vi "Store UI Ref.vi"(8 "error in (no error)":errorcluster, 11 "Mag Lab Measure Interface in":refnum<class "Mag Lab Measure UI.lvclass">) -> (0 "error out":errorcluster, 3 "Mag Lab Measure Interface out":refnum<class "Mag Lab Measure UI.lvclass">)   [LabVIEW 2015, in "Mag Lab Measure UI.lvclass"]
uses:
  Mag Lab Measure UI.lvclass
  Mag Lab Root/Mag Lab Root.lvclass/Mag Lab Root.ctl
  Mag Lab Measure UI.lvclass/Mag Lab Measure UI.ctl
  Mag Lab Root/Read Front Panel ref.vi
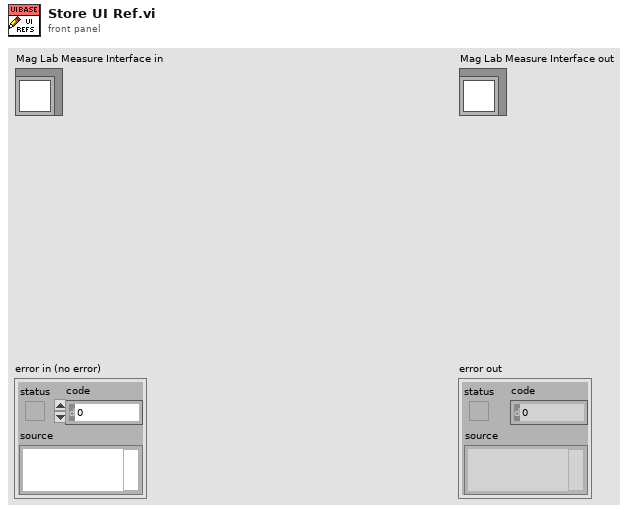
[diagram p1: front panel]
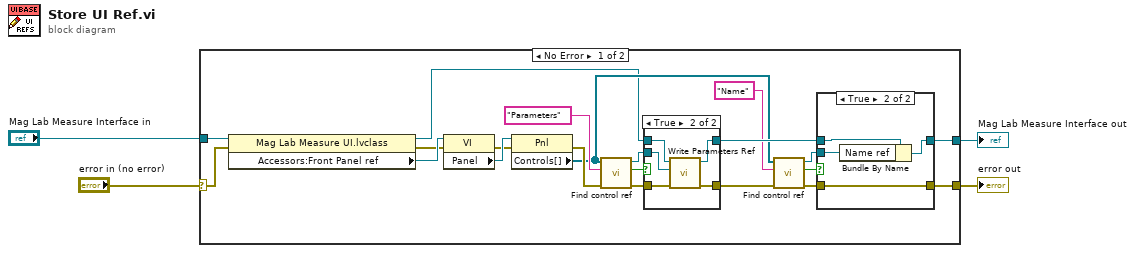
[diagram p0: block diagram]
diagram:
  n1 = case shown="No Error" "error in (no error)" {
    selector: "error in (no error)" -> [w5 w40]
    tunnel: [w16 w40] -> w3
    tunnel: [w17 w39] -> w1
    tunnel: "Mag Lab Measure Interface in" -> [w9 w39]
    frame No Error {
      n2 = property class="Mag Lab Measure UI.lvclass"(reference=w9, error in=w5) -> (reference out=w7:refnum<class "Mag Lab Measure UI.lvclass">, error out=w6:errorcluster, "Accessors:Front Panel ref"=w8:refnum<vi>)
      n3 = property class="VI"(reference=w8, error in=w6) -> (error out=w23:errorcluster, "Panel"=w24:refnum<vi>)  [unwired: 1 out]
      n4 = property class="Pnl"(reference=w24, error in=w23) -> (error out=w25:errorcluster, "Controls[]"=w11:refnum<vi>[])  [unwired: 1 out]
      n5 = call "Find control ref.vi"("error in (no error)"=w25, "Label"="Parameters", "Controls[]"=w11) -> ("error out"=w22:errorcluster, "Found"=w21:bool, "Control out"=w20:refnum<vi>)  [unwired: 6 in]
      n6 = case shown="True" w21 {
        tunnel: w7 -> [w33 w38]
        tunnel: [w33 w37] -> w18
        tunnel: w22 -> [w32 w36]
        tunnel: [w32 w35] -> w14
        tunnel: w20 -> [_ w34]
        frame False {
        }
        frame True {
          n7 = call "Write Parameters Ref.vi"("error in (no error)"=w36, "Parameters"=w34, "Mag Lab Measure Interface in"=w38) -> ("error out"=w35:errorcluster, "Mag Lab Measure Interface out"=w37:refnum<class "Mag Lab Measure UI.lvclass">)  [unwired: 7 in]
        }
      }
      n8 = call "Find control ref.vi"("error in (no error)"=w14, "Label"="Name", "Controls[]"=w11) -> ("error out"=w15:errorcluster, "Found"=w13:bool, "Control out"=w12:refnum<vi>)  [unwired: 6 in]
      n9 = case shown="True" w13 {
        tunnel: w18 -> [w27 w31]
        tunnel: [w27 w30] -> w17
        tunnel: w15 -> [w26 w28]
        tunnel: [w26 w28] -> w16
        tunnel: w12 -> [_ w29]
        frame False {
        }
        frame True {
          n10 = Bundle By Name(cluster=w31, "Name ref"=w29) -> (w30:refnum<class "Mag Lab Measure UI.lvclass">)
        }
      }
    }
    frame Error {
    }
  }
  "error out" <- w3
  "Mag Lab Measure Interface out" <- w1
